vi "ShoulderCmdSpecificAngle.vi"(8 "error in (no error)":errorcluster, 11 "SpecificAngle":dbl) -> (0 "error out":errorcluster)   [LabVIEW 2023]
uses:
  <vilib>/Rock Robotics/WPI/ThirdParty/JAS_Junk/TrajLib/VI/BoolCmd_Send_Internal.vi
  <vilib>/Rock Robotics/WPI/ThirdParty/JAS_Junk/TrajLib/VI/BoolCmd_ObtainQueue.vi
  Elevator/ElevatorGlobal.vi
  <vilib>/Rock Robotics/WPI/ThirdParty/JAS_Junk/TrajLib/Trajectory_Library.lvlib
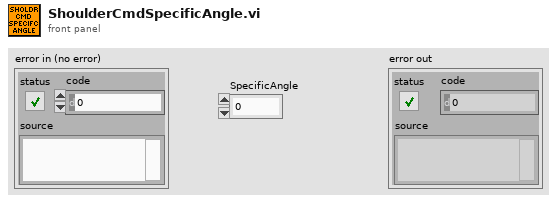
[diagram p1: front panel]
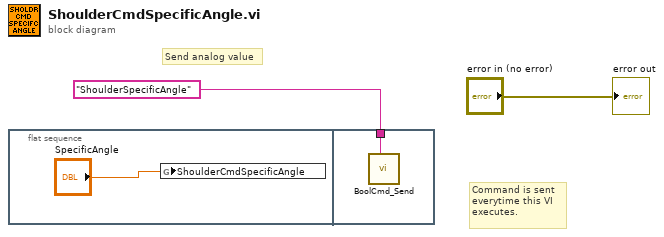
[diagram p0: block diagram]
diagram:
  # "Command is sent\neverytime this VI\nexecutes."
  # "Send analog value"
  n1 = flat-sequence {
    tunnel: "ShoulderSpecificAngle" ("Command Name") -> [w4]
    frame #0 {
      n2 = global write "ElevatorGlobal.vi" "ShoulderCmdSpecificAngle"("SpecificAngle") -> ()
    }
    frame #1 {
      n3 = call <vilib>:"BoolCmd_Send.vi"("Command Name"=w4) -> ()  [unwired: 10 in, 1 out]
    }
  }
  "error out" <- "error in (no error)"
